vi "Drive Controller.vi"(8 "error in":errorcluster) -> ()   [LabVIEW 2018]
doc: "This VI executes continuously carrying out the current operation and responding to updates or new operation requests. It will often contain the timing or control code that is difficult to place directly in TeleOp. This VI generally opens all sensors and motors and isolates the rest of the robot code from knowing implementation details of how the operations are carried out."
uses:
  <vilib>/Rock Robotics/WPI/Framework/Completion Status.ctl
  Drive Setpoints.ctl
  Drive Operations.ctl
  Dawgma Programming Library/Controls/PurePursuit/RobotNeededPathData.ctl
  <vilib>/Rock Robotics/WPI/ThirdParty/Phoenix-LabVIEW/Motor Controller/Controls/CTRE_Phoenix_MotorControl_VelocityMeasurementPeriod.ctl
  Logging/DataNames.ctl
  <vilib>/Rock Robotics/WPI/DriverStation/WPI_DriverStationRobotMode2.ctl
  <vilib>/Rock Robotics/WPI/ThirdParty/Phoenix-LabVIEW/Motor Controller/Controls/CTRE_Phoenix_MotorControl_ControlMode.ctl
  <extravilib>/ChannelInstances/Lossy Stream-c(dbl,dbl,dbl,dbl,dbl,c(dbl,dbl))/Write With Abort.vi
  <extravilib>/ChannelInstances/Lossy Stream-c(dbl,dbl,dbl,dbl,dbl,c(dbl,dbl))/Read With Abort.vi
  <extravilib>/ChannelInstances/Lossy Stream-c(dbl,dbl,dbl,dbl,dbl,c(dbl,dbl))/Endpoint.vi
  <extravilib>/ChannelInstances/Lossy Stream-c(dbl,dbl,dbl,dbl,dbl,c(dbl,dbl))/EndpointRead.vi
  <vilib>/Rock Robotics/WPI/ThirdParty/Sensors/navX/_Processing Loop/FRIC_navX_Internal_SPI_ProcessingLoop.vi
  <extravilib>/ChannelInstances/Lossy Stream-c(dbl,dbl,dbl,dbl,dbl,c(dbl,dbl))/Instantiate.vi
  <extravilib>/ChannelInstances/Lossy Stream-c(dbl,dbl,dbl,dbl,dbl,c(dbl,dbl))/)Channel.vi
  <resource>/ChannelSupport/_ChannelSupport/WaitIfNeeded.vi
  Configuration/Constants.vi
  <vilib>/Rock Robotics/WPI/ThirdParty/Phoenix-LabVIEW/Motor Controller/Get/CTRE_Phoenix_MotorController_GetVoltage.vi
  Framework/Robot Global Data.vi
  Drive Published Globals.vi
  <vilib>/Rock Robotics/Network Tables/NT Write Number.vi
  <vilib>/Rock Robotics/WPI/ThirdParty/Phoenix-LabVIEW/Motor Controller/Get/CTRE_Phoenix_MotorController_GetSelectedSensorData.vi
  <extravilib>/ChannelInstances/Lossy Stream-c(dbl,dbl,dbl,dbl,dbl,c(dbl,dbl)).lvlib
panel:
  out "Vel":dbl(graph)
  in  "Window Size":i32=8
  in  "Velocity Measurement Period":T1=20 items=["Period_1ms"=1, "Period_2ms"=2, "Period_5ms"=5, "Period_10ms"=10, "Period_20ms"=20, "Period_25ms"=25, "Period_50ms"=50, "Period_100ms"=100]
  out "Sensor Data":T2
  in  "Gains":T3={"FFV"=0.0088, "FFA"=0.0017, "Vel PID"={"P"=0.02, "I"=0.0, "D"=0.0}} {"Vel PID"."D" format="%.3f"; "Vel PID"."I" format="%.3f"; "Vel PID"."P" format="%.3f"}
  in  "Interactive Values":T4={"Operation"=enum."Reserve", "Left Setpoint"=0.0, "Right Setpoint"=0.0, "Duration"=0.0, "RobotNeededPathData"={"Path"=[], "MaxVel"=0.0, "MaxAccel"=0.0, "Backwards?"=FALSE, "PointSpacing"=0.0, "LookaheadDist"=0.0, "Speed/Curve"=1.8, "SlowDistanceAtEnd"=12.0, "SlowSpeed"=15.0, "MaxDeAccel"=0.0}, "Angle"=0.0, "Distance"=0.0} {"RobotNeededPathData"."SlowSpeed" format="%#_13g"; "RobotNeededPathData"."SlowDistanceAtEnd" format="%#_13g"; "RobotNeededPathData"."Speed/Curve" format="%#_13g"}
  in  "Buttons":cluster{"Execute Cmd":bool, "Abort Cmd":bool}
  out "Command Timing":cluster{"Start Time (ms)":u32, "Iterations":i32}
  out "Status":T7
  out "Current\nCmd":string
  # "Tip: The graph shows the motor setpoints. It may also be helpful to observe inputs and sensor values.\nYou may also want to display tuning or debugging controls."
  # "Interactive Command: You may fill in the settings for a command\nand schedule it with the Execute button. You can observe and abort\nany command while fine tuning the code for the controller."
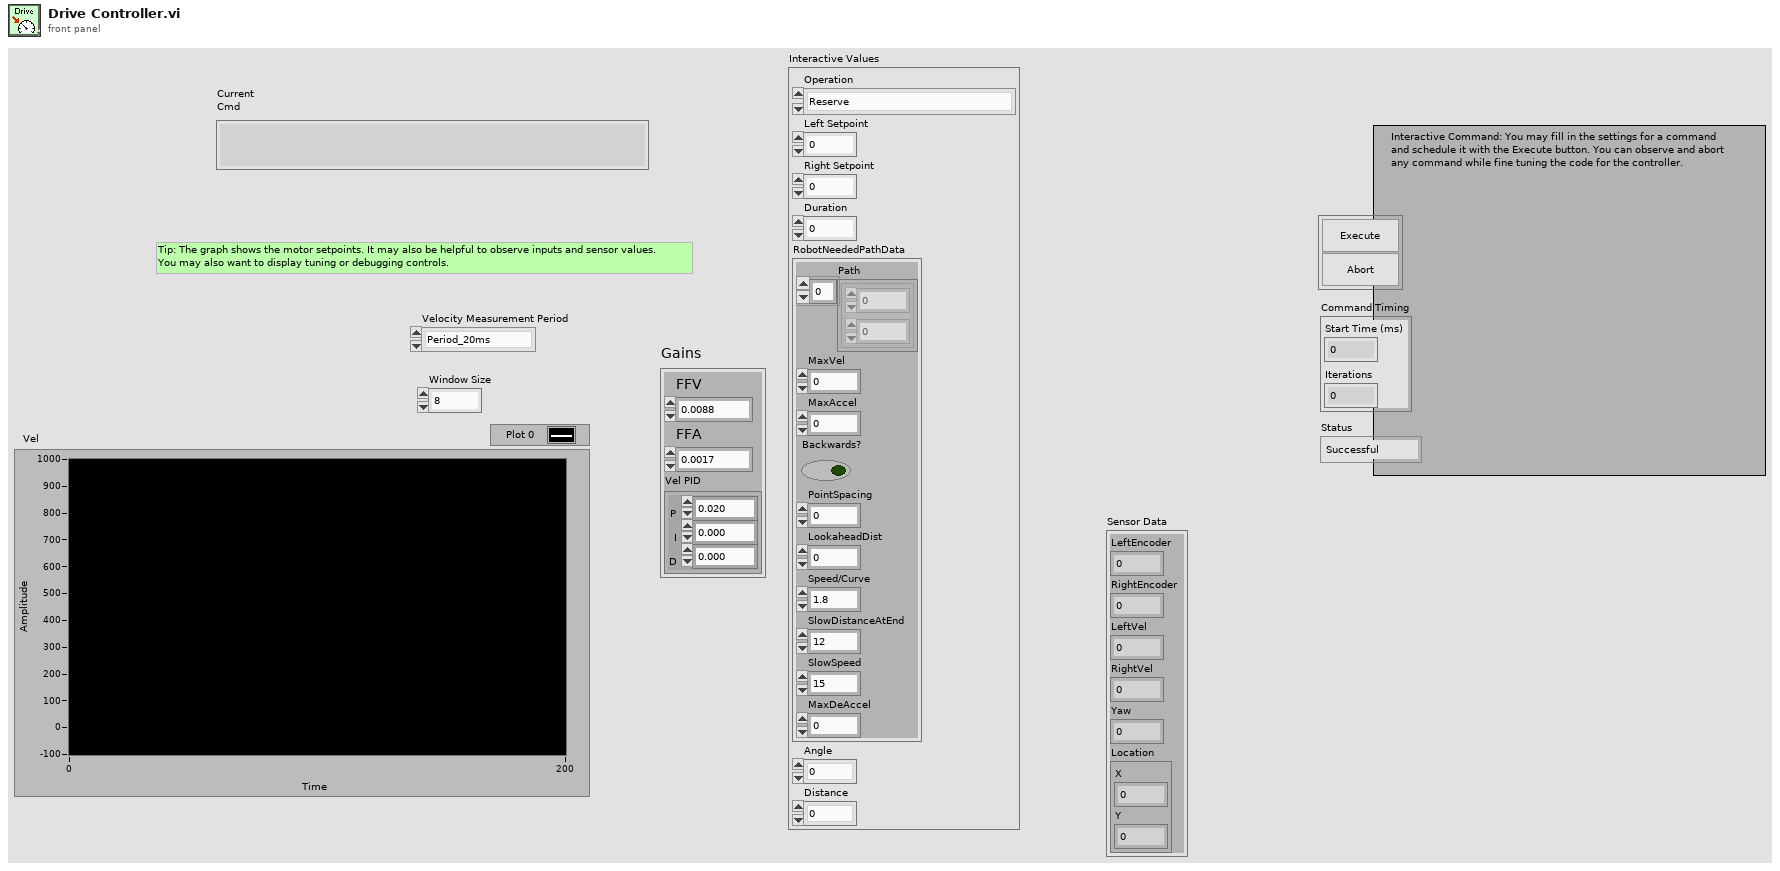
[diagram p1: front panel]
types:
  T1 = typedef "CTRE_Phoenix_MotorControl_VelocityMeasurementPeriod.ctl" = u16
  T2 = cluster{"LeftEncoder":dbl, "RightEncoder":dbl, "LeftVel":dbl, "RightVel":dbl, "Yaw":dbl, "Location":cluster{"X":dbl, "Y":dbl}}
  T3 = cluster{"FFV":dbl, "FFA":dbl, "Vel PID":cluster{"P":dbl, "I":dbl, "D":dbl}}
  T4 = typedef "Drive Setpoints.ctl" = cluster{"Operation":T5, "Left Setpoint":dbl, "Right Setpoint":dbl, "Duration":dbl, "RobotNeededPathData":T6, "Angle":dbl, "Distance":dbl}
  T5 = typedef "Drive Operations.ctl" = enum16{"Reserve", "Read Current", "Immediate", "Drive for Time", "Drive for Distance", "Drive Path", "Turn to Angle"}
  T6 = typedef "RobotNeededPathData.ctl" = cluster{"Path":cluster{dbl, dbl}[], "MaxVel":dbl, "MaxAccel":dbl, "Backwards?":bool, "PointSpacing":dbl, "LookaheadDist":dbl, "Speed/Curve":dbl, "SlowDistanceAtEnd":dbl, "SlowSpeed":dbl, "MaxDeAccel":dbl}
  T7 = typedef "Completion Status.ctl" = enum16{"Successful", "Aborted", "Incomplete"}
  T8 = typedef "Command Status Info.ctl" = cluster{"Name":string, "Status":T7, "notifier out":T9}
  T9 = typedef "Completion Notifier.ctl" = refnum<notifier>
  T10 = cluster{"SubSystem Data":T4, cluster{"Start Time (ms)":u32, "Iterations":i32}, cluster{"Command Info":T8, "Description":string, "Default Command":T4, "queue out":refnum<queue>, "Subsystem Name":string}}
  T11 = typedef "WPI_MotorControlDeviceRef.ctl" = cluster{"DeviceStatus":errorcluster, "Type":T12, "PWM":cluster{"PWM Channel":T13, "DeadBand":T14}, "CAN":cluster{"Device Number":u8, "SetOutput VI Ref":variant, "GetOutput VI Ref":variant, "Enable VI Ref":variant, "Disable VI Ref":variant, "Data":variant}, "Invert":bool, "DIO PWM":cluster{"PWM \"Enable\" Channel":T13, "DIOChannel":T15, "PWM Rate":dbl}}
  T12 = typedef "WPI_MotorControlType.ctl" = enum16{"PWM", "CAN", "DIO PWM"}
  T13 = typedef "FPGA_DIOPWMChannel.ctl" = enum8{"PWM 0", "PWM 1", "PWM 2", "PWM 3", "PWM 4", "PWM 5", "PWM 6", "PWM 7", "PWM 8", "PWM 9", "PWM MXP 0", "PWM MXP 1", "PWM MXP 2", "PWM MXP 3", "PWM MXP 4", "PWM MXP 5", "PWM MXP 6", "PWM MXP 7", "PWM MXP 8", "PWM MXP 9", "Invalid"}
  T14 = typedef "WPI_PWMDeadband.ctl" = cluster{"Name":string, "maxPositivePwm":i32, "minPositivePwm":i32, "centerPwm":i32, "maxNegativePwm":i32, "minNegativePwm":i32, "angularRange":u16}
  T15 = typedef "FPGA_DIOChannel.ctl" = enum8{"DIO 0", "DIO 1", "DIO 2", "DIO 3", "DIO 4", "DIO 5", "DIO 6", "DIO 7", "DIO 8", "DIO 9", "DIO MXP 0", "DIO MXP 1", "DIO MXP 2", "DIO MXP 3", "DIO MXP 4", "DIO MXP 5", "DIO MXP 6", "DIO MXP 7", "DIO MXP 8", "DIO MXP 9", "DIO MXP 10", "DIO MXP 11", "DIO MXP 12", "DIO MXP 13", "DIO MXP 14", "DIO MXP 15", "SPI Port CS1", "SPI Port CS2", "SPI Port CS3", "SPI Port MISO", "SPI Port MOSI", "Invalid"}
  T16 = typedef "DataNames.ctl" = enum16{"RobotMode", "FMSConnected", "DriveLeft", "DriveRight", "FloorHatchIntakeMotor", "SolenoidDirection", "EncoderLeft", "EncoderRight", "ArmEncoder", "ArmTopLimitSwitch", "ArmBottomLimitSwitch", "HatchLimitSwitch", "Yaw", "CheesyStraightJoystick", "CheesyTurnJoystick", "XCoordinate", "YCoordinate", "CPU", "DriveOperation", "Battery"}
  T17 = typedef "WPI_DriverStationRobotMode2.ctl" = enum16{"Autonomous Disabled", "Autonomous Enabled", "Teleop Disabled", "Teleop Enabled", "Disconnected", "Finish", "Test Disabled", "Test Enabled", "Emergency Stopped"}
  T18 = cluster{"Yaw":dbl, "Roll":dbl, "Pitch":dbl, "Heading":dbl, "Fused Heading":dbl}
  T19 = typedef "Lossy Stream-c(dbl,dbl,dbl,dbl,dbl,c(dbl,dbl)).lvlib/)Channel.ctl" = refnum<queue>
  T20 = cluster{"Yaw":dbl, "LeftEncoder":dbl, "LeftVel":dbl}
  T21 = enum16{"DemandType_Neutral", "DemandType_AuxPID", "DemandType_ArbitraryFeedForward"}
  T22 = typedef "CTRE_Phoenix_MotorControl_ControlMode.ctl" = u16
  T23 = cluster{"SubSystem Data":T4, cluster{"Start Time (ms)":u32, "Iterations":i32}, "Default Command Arguments":cluster{"Command Info":T8, "Description":string, "Default Command":T4, "queue out":refnum<queue>, "Subsystem Name":string}}
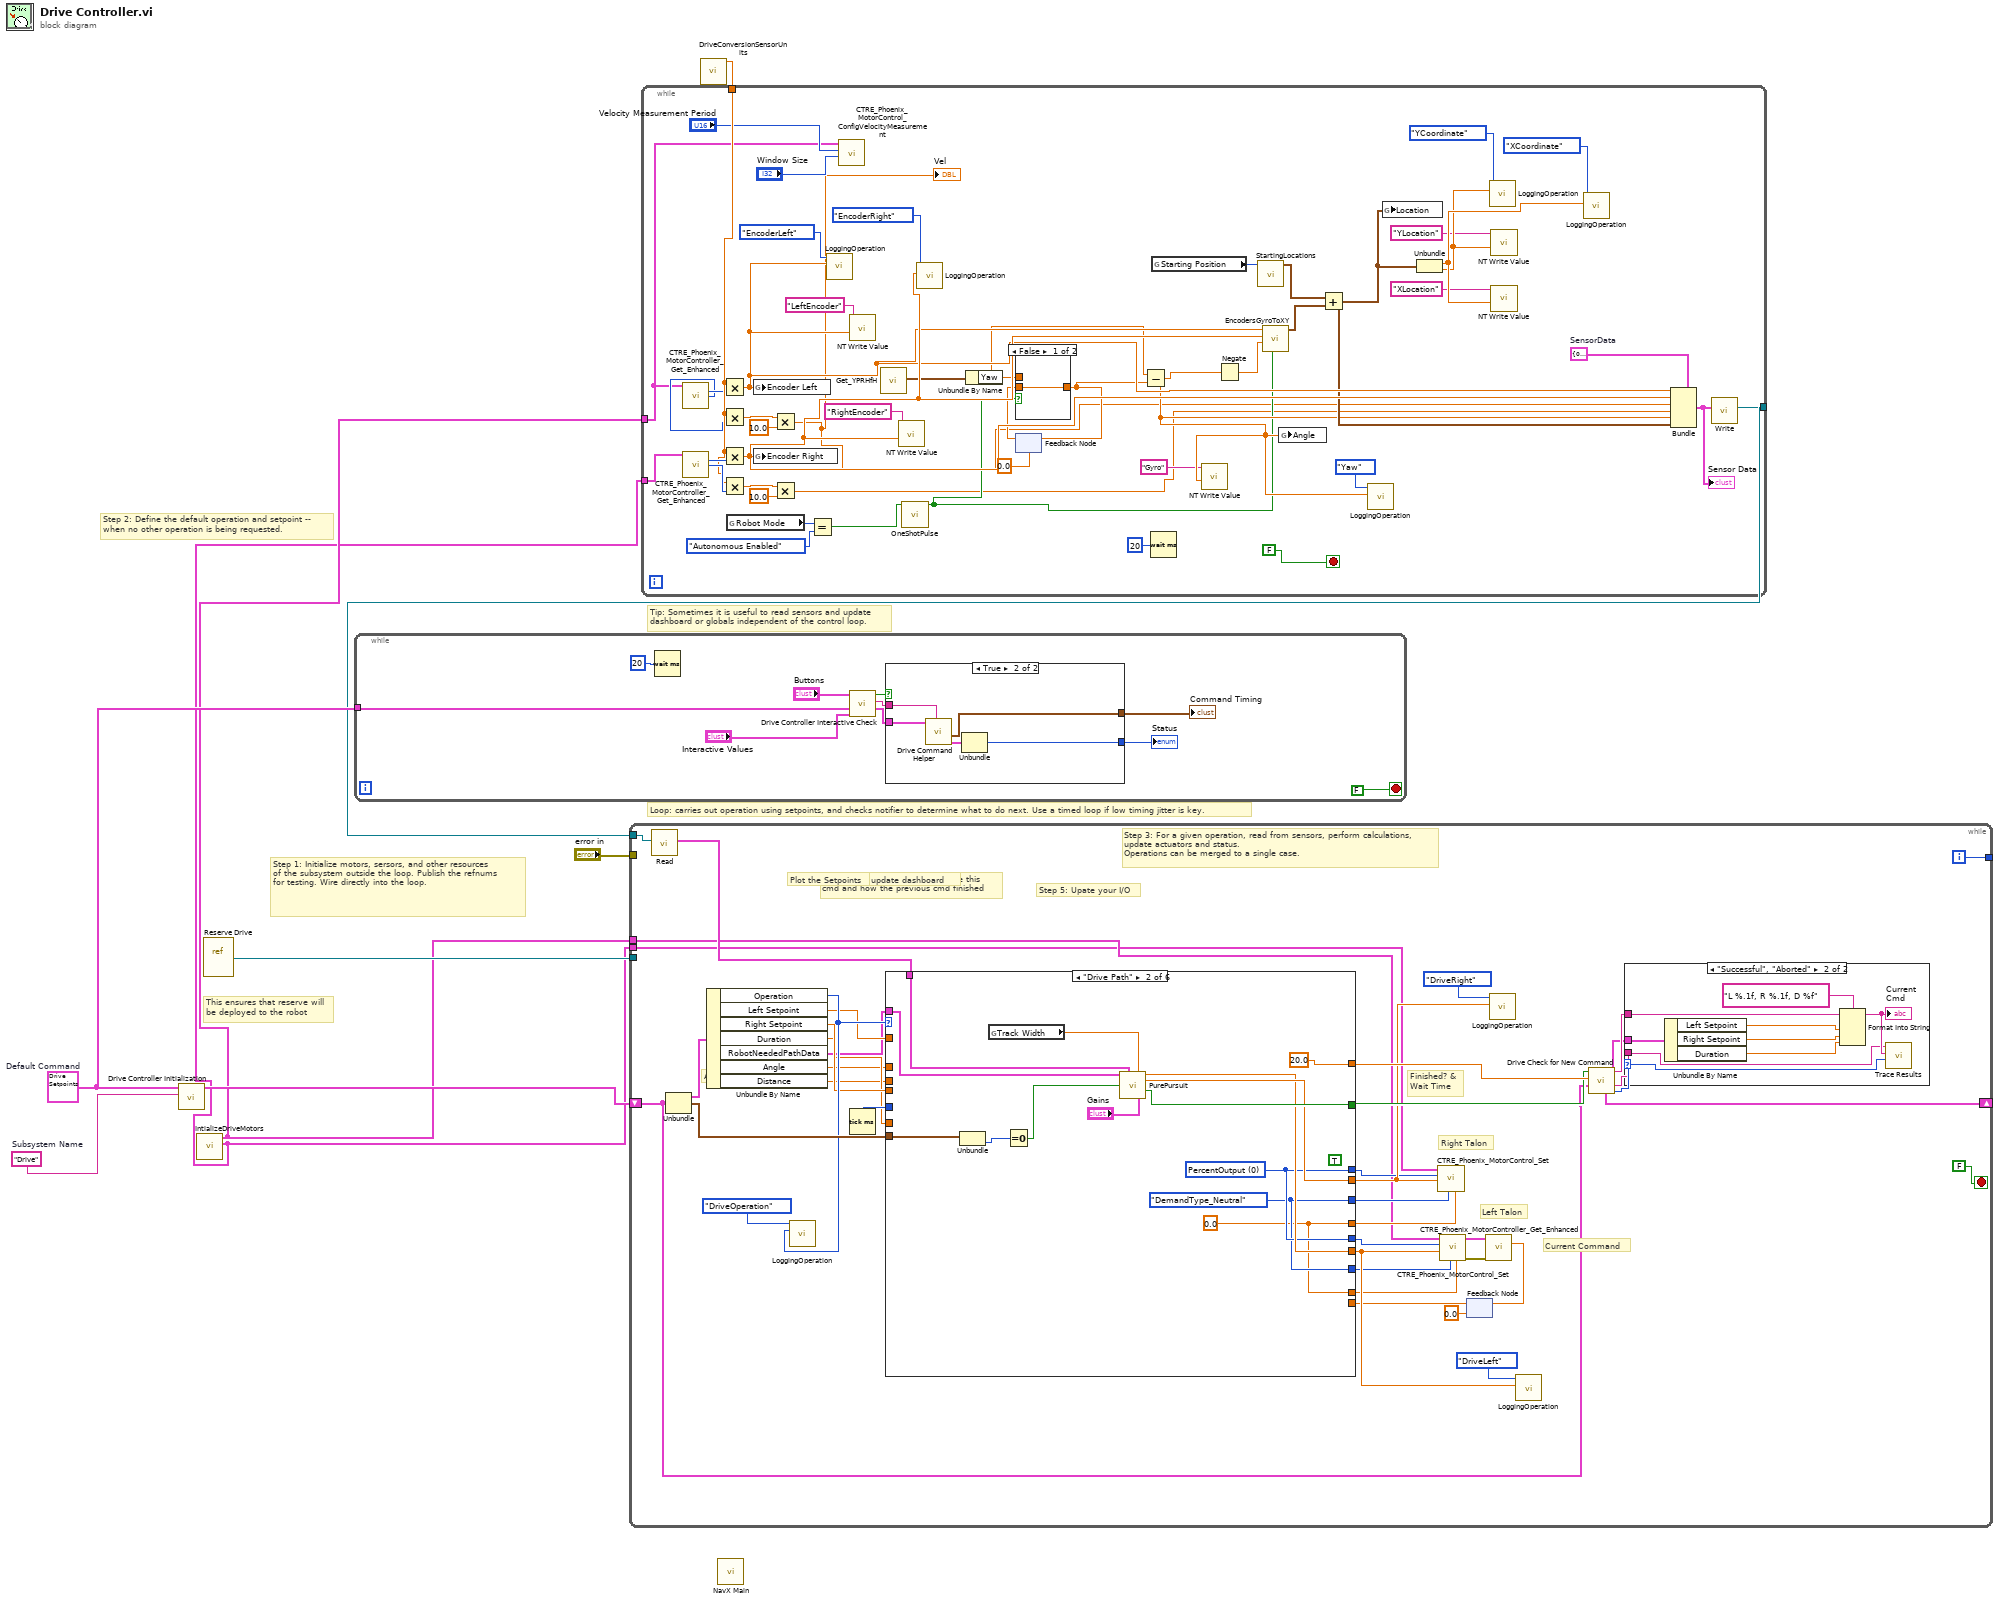
[diagram p0: block diagram]
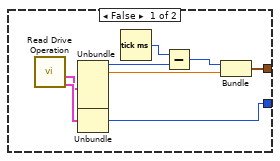
[diagram p3: hidden frame]
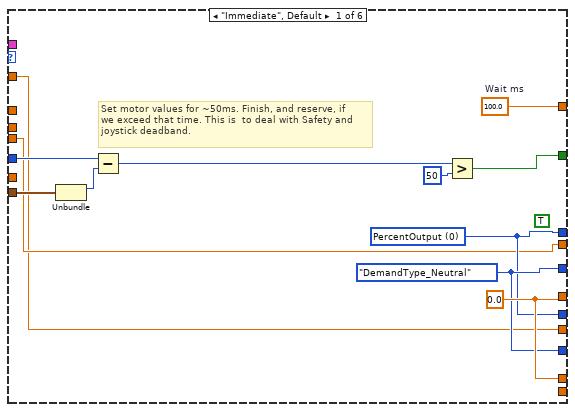
[diagram p4: hidden frame]
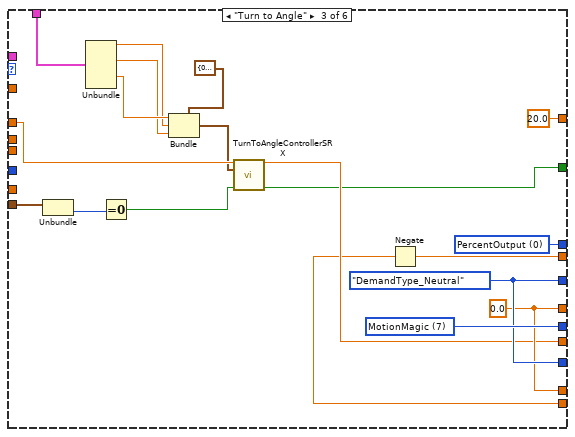
[diagram p5: hidden frame]
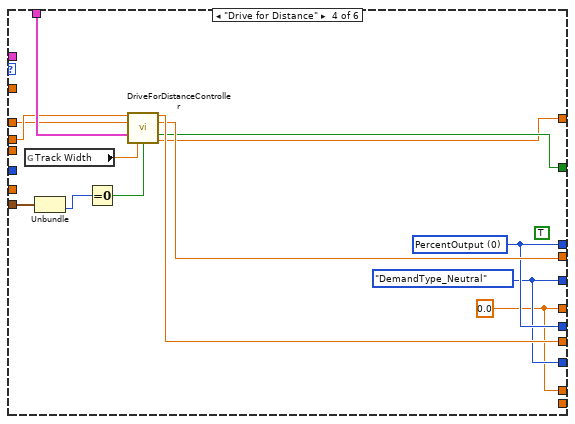
[diagram p6: hidden frame]
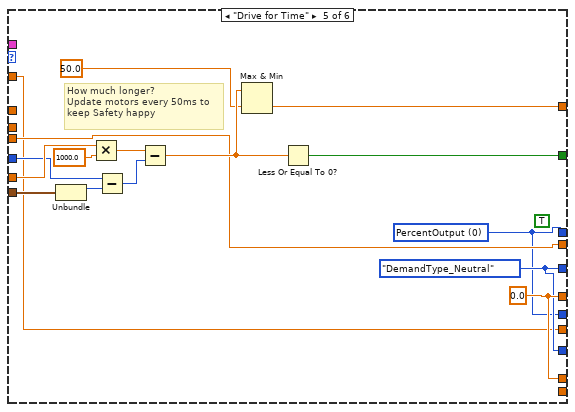
[diagram p7: hidden frame]
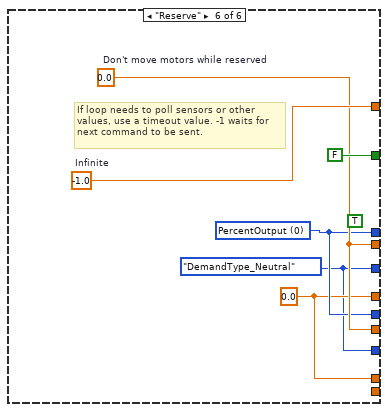
[diagram p8: hidden frame]
diagram:
  w5 = T4 {"Operation"=enum."Reserve", "Left Setpoint"=0.0, "Right Setpoint"=0.0, "Duration"=0.0, "RobotNeededPathData"={"Path"=[], "MaxVel"=0.0, "MaxAccel"=0.0, "Backwards?"=FALSE, "PointSpacing"=0.0, "LookaheadDist"=0.0, "Speed/Curve"=1.8, "SlowDistanceAtEnd"=12.0, "SlowSpeed"=15.0, "MaxDeAccel"=0.0}, "Angle"=0.0, "Distance"=0.0}  # Default Command
  w9 = "Drive"  # Subsystem Name
  # "Step 2: Define the default operation and setpoint --\nwhen no other operation is being requested."
  # "Step 1: Initialize motors, sersors, and other resources\nof the subsystem outside the loop. Publish the refnums\nfor testing. Wire directly into the loop."
  # "This ensures that reserve will\nbe deployed to the robot"
  # "Tip: Sometimes it is useful to read sensors and update\ndashboard or globals independent of the control loop."
  # "Loop: carries out operation using setpoints, and checks notifier to determine what to do next. Use a timed loop if low timing jitter is key."
  n1 = call "Drive Controller Initialization.vi"("Subsystem Name"=w9, "Default Command"=w5) -> ("Current Command"=w7:T10)  [unwired: 9 in]
  n2 = call "IntializeDriveMotors.vi"() -> ("Left Motor Reference"=w2:T11, "Right Motor Reference"=w1:T11)  [unwired: 9 in]
  n3 = vi-ref "Reserve Drive.vi"() -> (w6:refnum<vi>)
  n4 = while {
    tunnel: w5 -> [w11]
    stop <- FALSE stop-if-true
    n5 = Wait (ms)(milliseconds to wait=u32 20) -> ()  [unwired: 1 out]
    n6 = call "Drive Controller Interactive Check.vi"("Interactive Command In"="Interactive Values", "Default Command"=w11, "Buttons"="Buttons") -> ("Interactive Command Out"=w13:T4, "Trace String"=w14:string, "Schedule"=w15:bool)  [unwired: 6 in]
    n7 = case shown="True" w15 {
      tunnel: [w24 w32] -> w16
      tunnel: [w23 w28] -> w17
      tunnel: w14 -> [_ w30]
      tunnel: w13 -> [_ w29]
      frame False {
        n8 = call "Read Drive Operation.vi"() -> ("Command Info"=w21:T8, "SubSystem Data"=w20:T4)  [unwired: 9 in, 1 out]
        n9 = Unbundle(w20) -> ("Operation"=w25:T5, "Left Setpoint"=w22:dbl)  [unwired: 5 out]
        n10 = Unbundle(w21) -> ("Status"=w24:T7)  [unwired: 2 out]
        n11 = Tick Count (ms)() -> (millisecond timer value=w27:u32)
        n12 = Subtract(x=w27, y=w25) -> (x-y=w26:u32)
        n13 = Bundle(w26, "Left Setpoint"=w22) -> (w23:cluster{u32, "Left Setpoint":dbl})  [unwired: 1 in]
      }
      frame True {
        n14 = call "Drive Command Helper.vi"("Description"=w30, "SubSystem Data"=w29) -> ("Command Info Out"=w31:T8, "Command Timing"=w28:cluster{"Start Time (ms)":u32, "Iterations":i32})  [unwired: 7 in, 1 out]
        n15 = Unbundle(w31) -> ("Status"=w32:T7)  [unwired: 2 out]
      }
    }
    "Status" <- w16
    "Command Timing" <- w17
  }
  n16 = call "DriveConversionSensorUnits.vi"() -> ("Inches per Sensor Units"=w4:dbl)  [unwired: 11 in]
  n17 = while {
    tunnel: w1 -> [w81]
    tunnel: w2 -> [w34]
    tunnel: w4 -> [w77]
    tunnel: [w46] -> w3
    stop <- FALSE stop-if-true
    w47 = T2 {"LeftEncoder"=0.0, "RightEncoder"=0.0, "LeftVel"=0.0, "RightVel"=0.0, "Yaw"=0.0, "Location"={"X"=0.0, "Y"=0.0}}  # SensorData
    n18 = call-poly <vilib>:"CTRE_Phoenix_MotorController_Get_Enhanced.vi"("PhoenixMotorControlDevRef"=w34) -> ("Position (Raw Sensor Units)"=w75:i32, "Velocity (Raw Sensor Units per 100 ms)"=w74:i32)  [unwired: 11 in, 2 out]
    n19 = call-poly <vilib>:"CTRE_Phoenix_MotorController_Get_Enhanced.vi"("PhoenixMotorControlDevRef"=w81) -> ("Position (Raw Sensor Units)"=w80:i32, "Velocity (Raw Sensor Units per 100 ms)"=w79:i32)  [unwired: 11 in, 2 out]
    n20 = Multiply(x=w77, y=w75) -> (x*y=w73:dbl)
    n21 = Multiply(x=w77, y=w74) -> (x*y=w76:dbl)
    n22 = Multiply(x=w77, y=w80) -> (x*y=w78:dbl)
    n23 = Multiply(x=w77, y=w79) -> (x*y=w50:dbl)
    n24 = global read "Robot Global Data.vi" "Robot Mode"() -> (w58:T17)
    n25 = global write "Drive Published Globals.vi" "Encoder Left"(w73) -> ()
    n26 = global write "Drive Published Globals.vi" "Encoder Right"(w78) -> ()
    n27 = Multiply(x=w76, y=10.0 ("x*y")) -> (x*y=w33:dbl)
    "Vel" <- w33
    n28 = Multiply(x=w50, y=10.0 ("x*y")) -> (x*y=w51:dbl)
    n29 = Equal?(x=w58, y=WPI_DriverStationRobotMode2."Autonomous Enabled") -> (x = y?=w60:bool)
    n30 = call "LoggingOperation.vi"("Data"=w73, "Name"=DataNames."EncoderLeft") -> ()  [unwired: 9 in, 1 out]
    n31 = call <vilib>:"CTRE_Phoenix_MotorControl_ConfigVelocityMeasurement.vi"("Window Size"="Window Size", "Velocity Measurement Period"="Velocity Measurement Period", "PhoenixMotorControlDevRef"=w34) -> ()  [unwired: 7 in, 2 out]
    n32 = call-poly <vilib>:"NT Write Value.vi"("Numeric"=w73, "Name"="LeftEncoder") -> ()  [unwired: 9 in, 1 out]
    n33 = call <vilib>:"Get_YPRHfH.vi"() -> ("YRPHfH"=w63:T18)  [unwired: 11 in]
    n34 = call-poly <vilib>:"NT Write Value.vi"("Numeric"=w78, "Name"="RightEncoder") -> ()  [unwired: 9 in, 1 out]
    n35 = call "OneShotPulse.vi"("Input"=w60) -> ("Output"=w61:bool)  [unwired: 10 in]
    n36 = call "LoggingOperation.vi"("Data"=w78, "Name"=DataNames."EncoderRight") -> ()  [unwired: 9 in, 1 out]
    n37 = Unbundle By Name(w63) -> ("Yaw"=w64:dbl)
    n38 = feedback #1(0.0 ("Yaw")) -> (w66:dbl)
    n39 = case shown="False" w61 {
      tunnel: w64 -> [_ w83]
      tunnel: [w82 w83] -> w67
      tunnel: w66 -> [w82 _]
      frame False {
      }
      frame True {
      }
    }
    n40 = feedback-in #1(w67) -> ()
    n41 = Subtract(x=w64, y=w67) -> (x-y=w68:dbl)
    n42 = Wait (ms)(milliseconds to wait=u32 20) -> ()  [unwired: 1 out]
    n43 = global read "Robot Global Data.vi" "Starting Position"() -> (w56:i32)
    n44 = call-poly <vilib>:"NT Write Value.vi"("Numeric"=w68, "Name"="Gyro") -> ()  [unwired: 9 in, 1 out]
    n45 = Negate(x=w68) -> (-x=w69:dbl)
    n46 = call "StartingLocations.vi"("Index"=w56) -> ("Location"=w57:cluster{dbl, dbl})  [unwired: 10 in]
    n47 = call "EncodersGyroToXY.vi"("Reset"=w61, "Angle (degrees)"=w69, "Right Distance"=w78, "Left Distance"=w73) -> ("Location"=w70:cluster{dbl, dbl})  [unwired: 7 in]
    n48 = global write "Drive Published Globals.vi" "Angle"(w68) -> ()
    n49 = Add(x=w57, y=w70) -> (x+y=w71:cluster{dbl, dbl})
    n50 = call "LoggingOperation.vi"("Data"=w68, "Name"=DataNames."Yaw") -> ()  [unwired: 9 in, 1 out]
    n51 = global write "Drive Published Globals.vi" "Location"(w71) -> ()
    n52 = Unbundle(w71) -> (w55:dbl, w54:dbl)
    n53 = call "LoggingOperation.vi"("Data"=w54, "Name"=DataNames."YCoordinate") -> ()  [unwired: 9 in, 1 out]
    n54 = call-poly <vilib>:"NT Write Value.vi"("Numeric"=w54, "Name"="YLocation") -> ()  [unwired: 9 in, 1 out]
    n55 = call-poly <vilib>:"NT Write Value.vi"("Numeric"=w55, "Name"="XLocation") -> ()  [unwired: 9 in, 1 out]
    n56 = call "LoggingOperation.vi"("Data"=w55, "Name"=DataNames."XCoordinate") -> ()  [unwired: 9 in, 1 out]
    n57 = Bundle(cluster=w47, "LeftEncoder"=w73, "RightEncoder"=w78, "LeftVel"=w33, "RightVel"=w51, "Yaw"=w68, "Location"=w71) -> (w72:T2)
    "Sensor Data" <- w72
    n58 = call <extravilib>:"Write.vi"("element"=w72) -> ("channel"=w46:T19)  [unwired: 8 in, 2 out]
  }
  n59 = while {
    shift-right: [w119] -> _
    shift-left: w7 -> [w112]
    tunnel: [w122] -> _
    tunnel: "error in" -> [_]
    tunnel: w6 -> [_]
    tunnel: w3 -> [w105]
    tunnel: w1 -> [w92]
    tunnel: w2 -> [w93]
    i -> [w122]
    stop <- FALSE stop-if-true
    # "Right Talon"
    # "Left Talon"
    # "Step 5: Upate your I/O"
    # "Step 4: Format a string to describe this\ncmd and how the previous cmd finished"
    # "Current Command"
    # "Update motors and update dashboard"
    # "Plot the Setpoints"
    # "Access Cmd setpoints"
    # "Finished? &\nWait Time"
    # "Step 3: For a given operation, read from sensors, perform calculations,\nupdate actuators and status.\nOperations can be merged to a single case."
    n60 = call <extravilib>:"Read.vi"("channel"=w105) -> ("element"=w104:T2)  [unwired: 5 in, 5 out]
    n61 = Unbundle(w112) -> ("SubSystem Data"=w106:T4, w113:cluster{"Start Time (ms)":u32, "Iterations":i32})  [unwired: 1 out]
    n62 = Unbundle By Name(w106) -> ("Operation"=w111:T5, "Left Setpoint"=w110:dbl, "Right Setpoint"=w109:dbl, "Duration"=w108:dbl, "RobotNeededPathData"=w107:T6, "Angle"=w103:dbl, "Distance"=w94:dbl)
    n63 = call "LoggingOperation.vi"("Data"=w111, "Name"=DataNames."DriveOperation") -> ()  [unwired: 9 in, 1 out]
    n64 = Tick Count (ms)() -> (millisecond timer value=w121:u32)
    n65 = feedback #2(0.0 ("Output Current")) -> (w88:dbl)
    n66 = case shown="\"Drive Path\"" w111 {
      tunnel: [w135 20.0 20.0 ("Infinite") w170 w188 w204] -> w118
      tunnel: [w130 w148 w159 w171 w193 FALSE ("ignore previous (F)")] -> w117
      tunnel: w113 -> [w129 w144 w168 w179 w195 _]
      tunnel: [w125 w140 w157 w175 w187 w202] -> w101
      tunnel: [w124 w139 w161 w176 w183 w202] -> w102
      tunnel: w110 -> [w124 _ _ _ w183 _]
      tunnel: w109 -> [w125 _ _ _ w187 _]
      tunnel: w108 -> [_ _ _ _ w192 _]
      tunnel: w121 -> [w131 _ _ _ w191 _]
      tunnel: w107 -> [_ w149 _ _ _ _]
      tunnel: w104 -> [_ w147 w155 w182 _ _]
      tunnel: w103 -> [_ _ w166 w180 _ _]
      tunnel: [w126 w138 w164 w174 w184 w201] -> w100
      tunnel: [w127 w137 w163 w173 w185 w199] -> w99
      tunnel: [w128 w136 w162 w169 w186 w200] -> w98
      tunnel: [w126 w138 w156 w174 w184 w201] -> w97
      tunnel: [w127 w137 w163 w173 w185 w199] -> w96
      tunnel: [w128 w136 w162 w169 w186 w200] -> w95
      tunnel: w94 -> [_ _ _ w181 _ _]
      tunnel: w88 -> [_ _ w158 _ _ _]
      frame "Immediate", Default {
        (unwired) TRUE ("Done")
        w128 = 0.0 ("Demand1")
        w127 = T21."DemandType_Neutral" ("DemandType")
        w126 = T22 0 items=["PercentOutput"=0, "Position"=1, "Velocity"=2, "Current"=3, "Follower"=5, "MotionProfile"=6, "MotionMagic"=7, "MotionProfileArc"=10, "Disabled"=15] ("Control Mode")
        w135 = 100.0  # Wait ms
        # "Set motor values for ~50ms. Finish, and reserve, if\nwe exceed that time. This is  to deal with Safety and\njoystick deadband."
        n67 = Unbundle(w129) -> ("Start Time (ms)"=w132:u32)  [unwired: 1 out]
        n68 = Subtract(x=w131, y=w132) -> (x-y=w133:u32)
        n69 = Greater?(x=w133, y=u8 50 ("Left Motor")) -> (0:w130:bool)
      }
      frame "Drive Path" {
        (unwired) TRUE ("Done")
        w136 = 0.0 ("Demand1")
        w137 = T21."DemandType_Neutral" ("DemandType")
        w138 = T22 0 items=["PercentOutput"=0, "Position"=1, "Velocity"=2, "Current"=3, "Follower"=5, "MotionProfile"=6, "MotionMagic"=7, "MotionProfileArc"=10, "Disabled"=15] ("Control Mode")
        n70 = Unbundle(w144) -> ("Iterations"=w145:i32)  [unwired: 1 out]
        n71 = global read "Constants.vi" "Track Width"() -> (w142:dbl)
        n72 = Equal To 0?(x=w145) -> (x = 0?=w146:bool)
        n73 = call "PurePursuit.vi"("RobotNeededPathData"=w149, "SensorData"=w147, "Trackwidth"=w142, "Reset"=w146, "Gains"="Gains") -> ("LeftValue"=w139:dbl, "RightValue"=w140:dbl, "Done"=w148:bool)  [unwired: 5 in, 3 out]
      }
      frame "Turn to Angle" {
        w156 = T22 0 items=["PercentOutput"=0, "Position"=1, "Velocity"=2, "Current"=3, "Follower"=5, "MotionProfile"=6, "MotionMagic"=7, "MotionProfileArc"=10, "Disabled"=15] ("Control Mode")
        w162 = 0.0 ("Demand1")
        w163 = T21."DemandType_Neutral" ("DemandType")
        w164 = T22 7 items=["PercentOutput"=0, "Position"=1, "Velocity"=2, "Current"=3, "Follower"=5, "MotionProfile"=6, "MotionMagic"=7, "MotionProfileArc"=10, "Disabled"=15] ("Control Mode")
        n74 = Unbundle(w168) -> ("Iterations"=w167:i32)  [unwired: 1 out]
        n75 = Unbundle(w155) -> ("LeftEncoder"=w153:dbl, "LeftVel"=w152:dbl, "Yaw"=w154:dbl)  [unwired: 3 out]
        n76 = Equal To 0?(x=w167) -> (x = 0?=w165:bool)
        n77 = Bundle(cluster=T20 {"Yaw"=0.0, "LeftEncoder"=0.0, "LeftVel"=0.0}, "Yaw"=w154, "LeftEncoder"=w153, "LeftVel"=w152) -> (w151:T20)
        n78 = call "TurnToAngleControllerSRX.vi"("TargetAngle"=w166, "Robot"=w151, "Reset"=w165) -> ("TargetEncoderValue"=w161:dbl, "Done"=w159:bool)  [unwired: 7 in, 4 out]
        n79 = Negate(x=w158) -> (-x=w157:dbl)
      }
      frame "Drive for Distance" {
        (unwired) TRUE ("Done")
        w169 = 0.0 ("Demand1")
        w173 = T21."DemandType_Neutral" ("DemandType")
        w174 = T22 0 items=["PercentOutput"=0, "Position"=1, "Velocity"=2, "Current"=3, "Follower"=5, "MotionProfile"=6, "MotionMagic"=7, "MotionProfileArc"=10, "Disabled"=15] ("Control Mode")
        n80 = global read "Constants.vi" "Track Width"() -> (w172:dbl)
        n81 = Unbundle(w179) -> ("Iterations"=w178:i32)  [unwired: 1 out]
        n82 = Equal To 0?(x=w178) -> (x = 0?=w177:bool)
        n83 = call "DriveForDistanceController.vi"("Distance"=w181, "Angle"=w180, "SensorData"=w182, "Trackwidth"=w172, "Reset"=w177) -> ("Left Speed"=w176:dbl, "Right Speed"=w175:dbl, "Done"=w171:bool, "Time Left"=w170:dbl)  [unwired: 6 in, 1 out]
      }
      frame "Drive for Time" {
        (unwired) TRUE ("Done")
        w186 = 0.0 ("Demand1")
        w185 = T21."DemandType_Neutral" ("DemandType")
        w184 = T22 0 items=["PercentOutput"=0, "Position"=1, "Velocity"=2, "Current"=3, "Follower"=5, "MotionProfile"=6, "MotionMagic"=7, "MotionProfileArc"=10, "Disabled"=15] ("Control Mode")
        # "How much longer?\nUpdate motors every 50ms to\nkeep Safety happy"
        n84 = Unbundle(w195) -> ("Start Time (ms)"=w194:u32)  [unwired: 1 out]
        n85 = Multiply(x=w192, y=1000.0) -> (x*y=w197:dbl)
        n86 = Subtract(x=w191, y=w194) -> (x-y=w198:u32)
        n87 = Subtract(x=w197, y=w198) -> (x-y=w190:dbl)
        n88 = Max & Min(x=w190, y=50.0) -> (min(x,y)=w188:dbl)  [unwired: 1 out]
        n89 = Less Or Equal To 0?(x=w190) -> (x <= 0?=w193:bool)
      }
      frame "Reserve" {
        (unwired) TRUE ("Done")
        w199 = T21."DemandType_Neutral" ("DemandType")
        w200 = 0.0 ("Demand1")
        w201 = T22 0 items=["PercentOutput"=0, "Position"=1, "Velocity"=2, "Current"=3, "Follower"=5, "MotionProfile"=6, "MotionMagic"=7, "MotionProfileArc"=10, "Disabled"=15] ("Control Mode")
        w202 = 0.0  # Don't move motors while reserved
        w204 = -1.0  # Infinite
        # "If loop needs to poll sensors or other\nvalues, use a timeout value. -1 waits for\nnext command to be sent."
      }
    }
    n90 = call <vilib>:"CTRE_Phoenix_MotorControl_Set.vi"("Demand1"=w95, "DemandType"=w96, "Output"=w101, "Control Mode"=w97, "PhoenixMotorControlDevRef"=w92) -> ()  [unwired: 5 in, 2 out]
    n91 = call <vilib>:"CTRE_Phoenix_MotorControl_Set.vi"("Demand1"=w98, "DemandType"=w99, "Output"=w102, "Control Mode"=w100, "PhoenixMotorControlDevRef"=w93) -> ("error out"=w90:errorcluster, "PhoenixMotorControlDevRef"=w91:T11)  [unwired: 5 in]
    n92 = call-poly <vilib>:"CTRE_Phoenix_MotorController_Get_Enhanced.vi"("PhoenixMotorControlDevRef"=w91, "error in"=w90) -> ("Percent Output"=w89:dbl)  [unwired: 9 in, 4 out]
    n93 = feedback-in #2(w89) -> ()
    n94 = call "LoggingOperation.vi"("Data"=w101, "Name"=DataNames."DriveRight") -> ()  [unwired: 9 in, 1 out]
    n95 = call "LoggingOperation.vi"("Data"=w102, "Name"=DataNames."DriveLeft") -> ()  [unwired: 9 in, 1 out]
    n96 = call "Drive Check for New Command.vi"("input cluster"=w112, "Wait time (ms)"=w118, "Finished?"=w117) -> ("Completion"=w120:T7, "Subsystem Name"=w114:string, "Current Command"=w115:T4, "Initial Trace String"=w116:string, "Next Command"=w119:T23)  [unwired: 4 in]
    n97 = case shown="\"Successful\", \"Aborted\"" w120 {
      selector: w120 -> [_ w213]
      tunnel: w116 -> [_ w208]
      tunnel: w115 -> [_ w209]
      tunnel: w114 -> [_ w205]
      frame "Incomplete", Default {
        # "Continuing current command"
      }
      frame "Successful", "Aborted" {
        # "Report and setup for next command"
        n98 = Unbundle By Name(w209) -> ("Left Setpoint"=w211:dbl, "Right Setpoint"=w212:dbl, "Duration"=w206:dbl)
        n99 = Format Into String(format string="L %.1f, R %.1f, D %f", initial string=w208, w211, w212, w206) -> (resulting string=w207:string)  [unwired: 1 in, 1 out]
        "Current\nCmd" <- w207
        n100 = call <vilib>:"Trace Results.vi"("Status of previous command"=w213, "Description"=w207, "Subsystem"=w205) -> ()  [unwired: 9 in]
      }
    }
  }
  n101 = call-poly <vilib>:"NavX Main.vi"() -> ()  [unwired: 12 in]
